vi "Drums with Guitar.vi"() -> ()   [LabVIEW 2009]
uses:
  <vilib>/vision/Image Controls.llb/IMAQ Image.ctl
  <vilib>/Instr/_visa.llb/VISA Configure Serial Port (Instr).vi
  <vilib>/Analysis/3filter.llb/Filter Passband Type.ctl
  <vilib>/Analysis/3filter.llb/Butterworth Filter (DBL).vi
  <vilib>/vision/NI_Vision_Development_Module.lvlib
  <vilib>/Analysis/NI_AALBase.lvlib
panel:
  in  "Orange Guitar":T1={"Global Rectangle"=[220, 296, 225, 371], "Contours"=[{"ID"=enum."External", "Type"=2, "Coordinates"=[224, 370, 220, 296]}]} {"Contours"."Type" items=["No Selection", "Point", "Line", "Rectangle", "Oval", "Polygon", "Freehand Region", "Annulus", "Unused2", "Unused3", "Broken Line", "Freehand Line", "Rotated Rectangle"]}
  out "Orange Guitar":dbl[](graph)
  out "Orange Guitar LED":bool
  in  "sampling 8":dbl=1.0 format="%0.2f"
  in  "high 9":dbl=60.0 format="%0.2f"
  in  "low  8":dbl=0.12500000000000006 format="%0.4f"
  out "Orange Guitar":T1={"Global Rectangle"=[300, 297, 320, 380], "Contours"=[{"ID"=enum."External", "Type"=2, "Coordinates"=[300, 379, 319, 297]}]} {"Contours"."Type" items=["No Selection", "Point", "Line", "Rectangle", "Oval", "Polygon", "Freehand Region", "Annulus", "Unused2", "Unused3", "Broken Line", "Freehand Line", "Rotated Rectangle"]}
  in  "Green Guitar":T1={"Global Rectangle"=[100, 292, 131, 371], "Contours"=[{"ID"=enum."External", "Type"=2, "Coordinates"=[100, 370, 130, 292]}]} {"Contours"."Type" items=["No Selection", "Point", "Line", "Rectangle", "Oval", "Polygon", "Freehand Region", "Annulus", "Unused2", "Unused3", "Broken Line", "Freehand Line", "Rotated Rectangle"]}
  in  "Blue Guitar":T1={"Global Rectangle"=[193, 293, 199, 374], "Contours"=[{"ID"=enum."External", "Type"=2, "Coordinates"=[193, 373, 198, 293]}]} {"Contours"."Type" items=["No Selection", "Point", "Line", "Rectangle", "Oval", "Polygon", "Freehand Region", "Annulus", "Unused2", "Unused3", "Broken Line", "Freehand Line", "Rotated Rectangle"]}
  in  "Red Guitar":T1={"Global Rectangle"=[129, 294, 154, 376], "Contours"=[{"ID"=enum."External", "Type"=2, "Coordinates"=[129, 375, 153, 294]}]} {"Contours"."Type" items=["No Selection", "Point", "Line", "Rectangle", "Oval", "Polygon", "Freehand Region", "Annulus", "Unused2", "Unused3", "Broken Line", "Freehand Line", "Rotated Rectangle"]}
  in  "Yellow Guitar":T1={"Global Rectangle"=[160, 295, 175, 378], "Contours"=[{"ID"=enum."External", "Type"=2, "Coordinates"=[160, 377, 174, 295]}]} {"Contours"."Type" items=["No Selection", "Point", "Line", "Rectangle", "Oval", "Polygon", "Freehand Region", "Annulus", "Unused2", "Unused3", "Broken Line", "Freehand Line", "Rotated Rectangle"]}
  in  "sampling  8":dbl=1.0 format="%0.2f"
  in  "high 8":dbl=60.0 format="%0.2f"
  out "Blue Guitar":dbl[](graph)
  in  "low 2":dbl=0.12500000000000006 format="%0.4f"
  out "Yellow Guitar":dbl[](graph)
  out "Yellow Guitar LED":bool
  in  "sampling 7":dbl=1.0 format="%0.2f"
  in  "high 7":dbl=60.0 format="%0.2f"
  in  "low  7":dbl=0.12500000000000006 format="%0.4f"
  out "Yellow Guitar":T1={"Global Rectangle"=[243, 262, 261, 384], "Contours"=[{"ID"=enum."External", "Type"=2, "Coordinates"=[260, 383, 243, 262]}]} {"Contours"."Type" items=["No Selection", "Point", "Line", "Rectangle", "Oval", "Polygon", "Freehand Region", "Annulus", "Unused2", "Unused3", "Broken Line", "Freehand Line", "Rotated Rectangle"]}
  out "Blue Guitar":T1={"Global Rectangle"=[168, 264, 180, 378], "Contours"=[{"ID"=enum."External", "Type"=2, "Coordinates"=[168, 377, 179, 264]}]} {"Contours"."Type" items=["No Selection", "Point", "Line", "Rectangle", "Oval", "Polygon", "Freehand Region", "Annulus", "Unused2", "Unused3", "Broken Line", "Freehand Line", "Rotated Rectangle"]}
  out "Green Guitar":dbl[](graph)
  out "Green Guitar LED":bool
  in  "sampling 6":dbl=1.0 format="%0.2f"
  in  "high 6":dbl=60.0 format="%0.2f"
  in  "low  6":dbl=0.12500000000000006 format="%0.4f"
  out "Green Guitar":T1={"Global Rectangle"=[406, 309, 423, 383], "Contours"=[{"ID"=enum."External", "Type"=2, "Coordinates"=[422, 382, 406, 309]}]} {"Contours"."Type" items=["No Selection", "Point", "Line", "Rectangle", "Oval", "Polygon", "Freehand Region", "Annulus", "Unused2", "Unused3", "Broken Line", "Freehand Line", "Rotated Rectangle"]}
  out "Red Guitar":dbl[](graph)
  out "Red Guitar LED":bool
  in  "sampling 5":dbl=1.0 format="%0.2f"
  in  "high 5":dbl=60.0 format="%0.2f"
  in  "low  5":dbl=0.12500000000000006 format="%0.4f"
  out "Red Guitar":T1={"Global Rectangle"=[300, 297, 320, 380], "Contours"=[{"ID"=enum."External", "Type"=2, "Coordinates"=[300, 379, 319, 297]}]} {"Contours"."Type" items=["No Selection", "Point", "Line", "Rectangle", "Oval", "Polygon", "Freehand Region", "Annulus", "Unused2", "Unused3", "Broken Line", "Freehand Line", "Rotated Rectangle"]}
  out "Blue Guitar LED":bool
  in  "Mask":T1 {"Contours"."Type" items=["No Selection", "Point", "Line", "Rectangle", "Oval", "Polygon", "Freehand Region", "Annulus", "Unused2", "Unused3", "Broken Line", "Freehand Line", "Rotated Rectangle"]}
  out "Image 2":T2(plugin-control)
  out "Red Line":T1={"Global Rectangle"=[300, 297, 320, 380], "Contours"=[{"ID"=enum."External", "Type"=2, "Coordinates"=[300, 379, 319, 297]}]} {"Contours"."Type" items=["No Selection", "Point", "Line", "Rectangle", "Oval", "Polygon", "Freehand Region", "Annulus", "Unused2", "Unused3", "Broken Line", "Freehand Line", "Rotated Rectangle"]}
  in  "Red Line":T1={"Global Rectangle"=[300, 297, 320, 380], "Contours"=[{"ID"=enum."External", "Type"=2, "Coordinates"=[300, 379, 319, 297]}]} {"Contours"."Type" items=["No Selection", "Point", "Line", "Rectangle", "Oval", "Polygon", "Freehand Region", "Annulus", "Unused2", "Unused3", "Broken Line", "Freehand Line", "Rotated Rectangle"]}
  out "Waveform Red":dbl[](graph)
  out "LED Red":bool
  in  "sampling 4":dbl=1.0 format="%0.2f"
  in  "high 4":dbl=60.0 format="%0.2f"
  in  "low  4":dbl=0.12500000000000006 format="%0.4f"
  out "Green Line":T1={"Global Rectangle"=[406, 309, 423, 383], "Contours"=[{"ID"=enum."External", "Type"=2, "Coordinates"=[422, 382, 406, 309]}]} {"Contours"."Type" items=["No Selection", "Point", "Line", "Rectangle", "Oval", "Polygon", "Freehand Region", "Annulus", "Unused2", "Unused3", "Broken Line", "Freehand Line", "Rotated Rectangle"]}
  in  "Blue Line":T1={"Global Rectangle"=[374, 278, 383, 377], "Contours"=[{"ID"=enum."External", "Type"=2, "Coordinates"=[382, 376, 374, 278]}]} {"Contours"."Type" items=["No Selection", "Point", "Line", "Rectangle", "Oval", "Polygon", "Freehand Region", "Annulus", "Unused2", "Unused3", "Broken Line", "Freehand Line", "Rotated Rectangle"]}
  in  "Green Line":T1={"Global Rectangle"=[406, 309, 423, 383], "Contours"=[{"ID"=enum."External", "Type"=2, "Coordinates"=[422, 382, 406, 309]}]} {"Contours"."Type" items=["No Selection", "Point", "Line", "Rectangle", "Oval", "Polygon", "Freehand Region", "Annulus", "Unused2", "Unused3", "Broken Line", "Freehand Line", "Rotated Rectangle"]}
  in  "low  3":dbl=0.12500000000000006 format="%0.4f"
  out "Waveform Green":dbl[](graph)
  out "LED Green":bool
  in  "sampling 3":dbl=1.0 format="%0.2f"
  in  "high 3":dbl=60.0 format="%0.2f"
  in  "Yellow Line":T1={"Global Rectangle"=[342, 292, 349, 377], "Contours"=[{"ID"=enum."External", "Type"=2, "Coordinates"=[342, 376, 348, 292]}]} {"Contours"."Type" items=["No Selection", "Point", "Line", "Rectangle", "Oval", "Polygon", "Freehand Region", "Annulus", "Unused2", "Unused3", "Broken Line", "Freehand Line", "Rotated Rectangle"]}
  out "Blue Line":T1={"Global Rectangle"=[168, 264, 180, 378], "Contours"=[{"ID"=enum."External", "Type"=2, "Coordinates"=[168, 377, 179, 264]}]} {"Contours"."Type" items=["No Selection", "Point", "Line", "Rectangle", "Oval", "Polygon", "Freehand Region", "Annulus", "Unused2", "Unused3", "Broken Line", "Freehand Line", "Rotated Rectangle"]}
  out "cluster":T3
  in  "baud rate (9600)":u32=9600
  in  "VISA resource name":refnum<visa-resource-name>
  out "number":u32
  out "decimal integer string":string
  out "Image Dst Out":T2
  out "Yellow Line":T1={"Global Rectangle"=[243, 262, 261, 384], "Contours"=[{"ID"=enum."External", "Type"=2, "Coordinates"=[260, 383, 243, 262]}]} {"Contours"."Type" items=["No Selection", "Point", "Line", "Rectangle", "Oval", "Polygon", "Freehand Region", "Annulus", "Unused2", "Unused3", "Broken Line", "Freehand Line", "Rotated Rectangle"]}
  in  "low  2":dbl=0.12500000000000006 format="%0.4f"
  in  "high 2":dbl=60.0 format="%0.2f"
  in  "sampling 2":dbl=1.0 format="%0.2f"
  out "LED Yellow":bool
  out "Waveform Yellow":dbl[](graph)
  in  "playtime":dbl=30.0
  out "Frame Number":i32
  in  "Frame Start":i32=2400
  out "Blue Drum":bool
  in  "low":dbl=0.12500000000000006 format="%0.4f"
  out "Blue Drum":dbl[](graph)
  in  "high":dbl=60.0 format="%0.2f"
  in  "sampling":dbl=1.0 format="%0.2f"
  in  "stop":bool
  in  "AVI Path":path
  # "BLUE"
  # "YELLOW"
  # "GREEN"
  # "RED"
  # "Drums"
  # "Guitar"
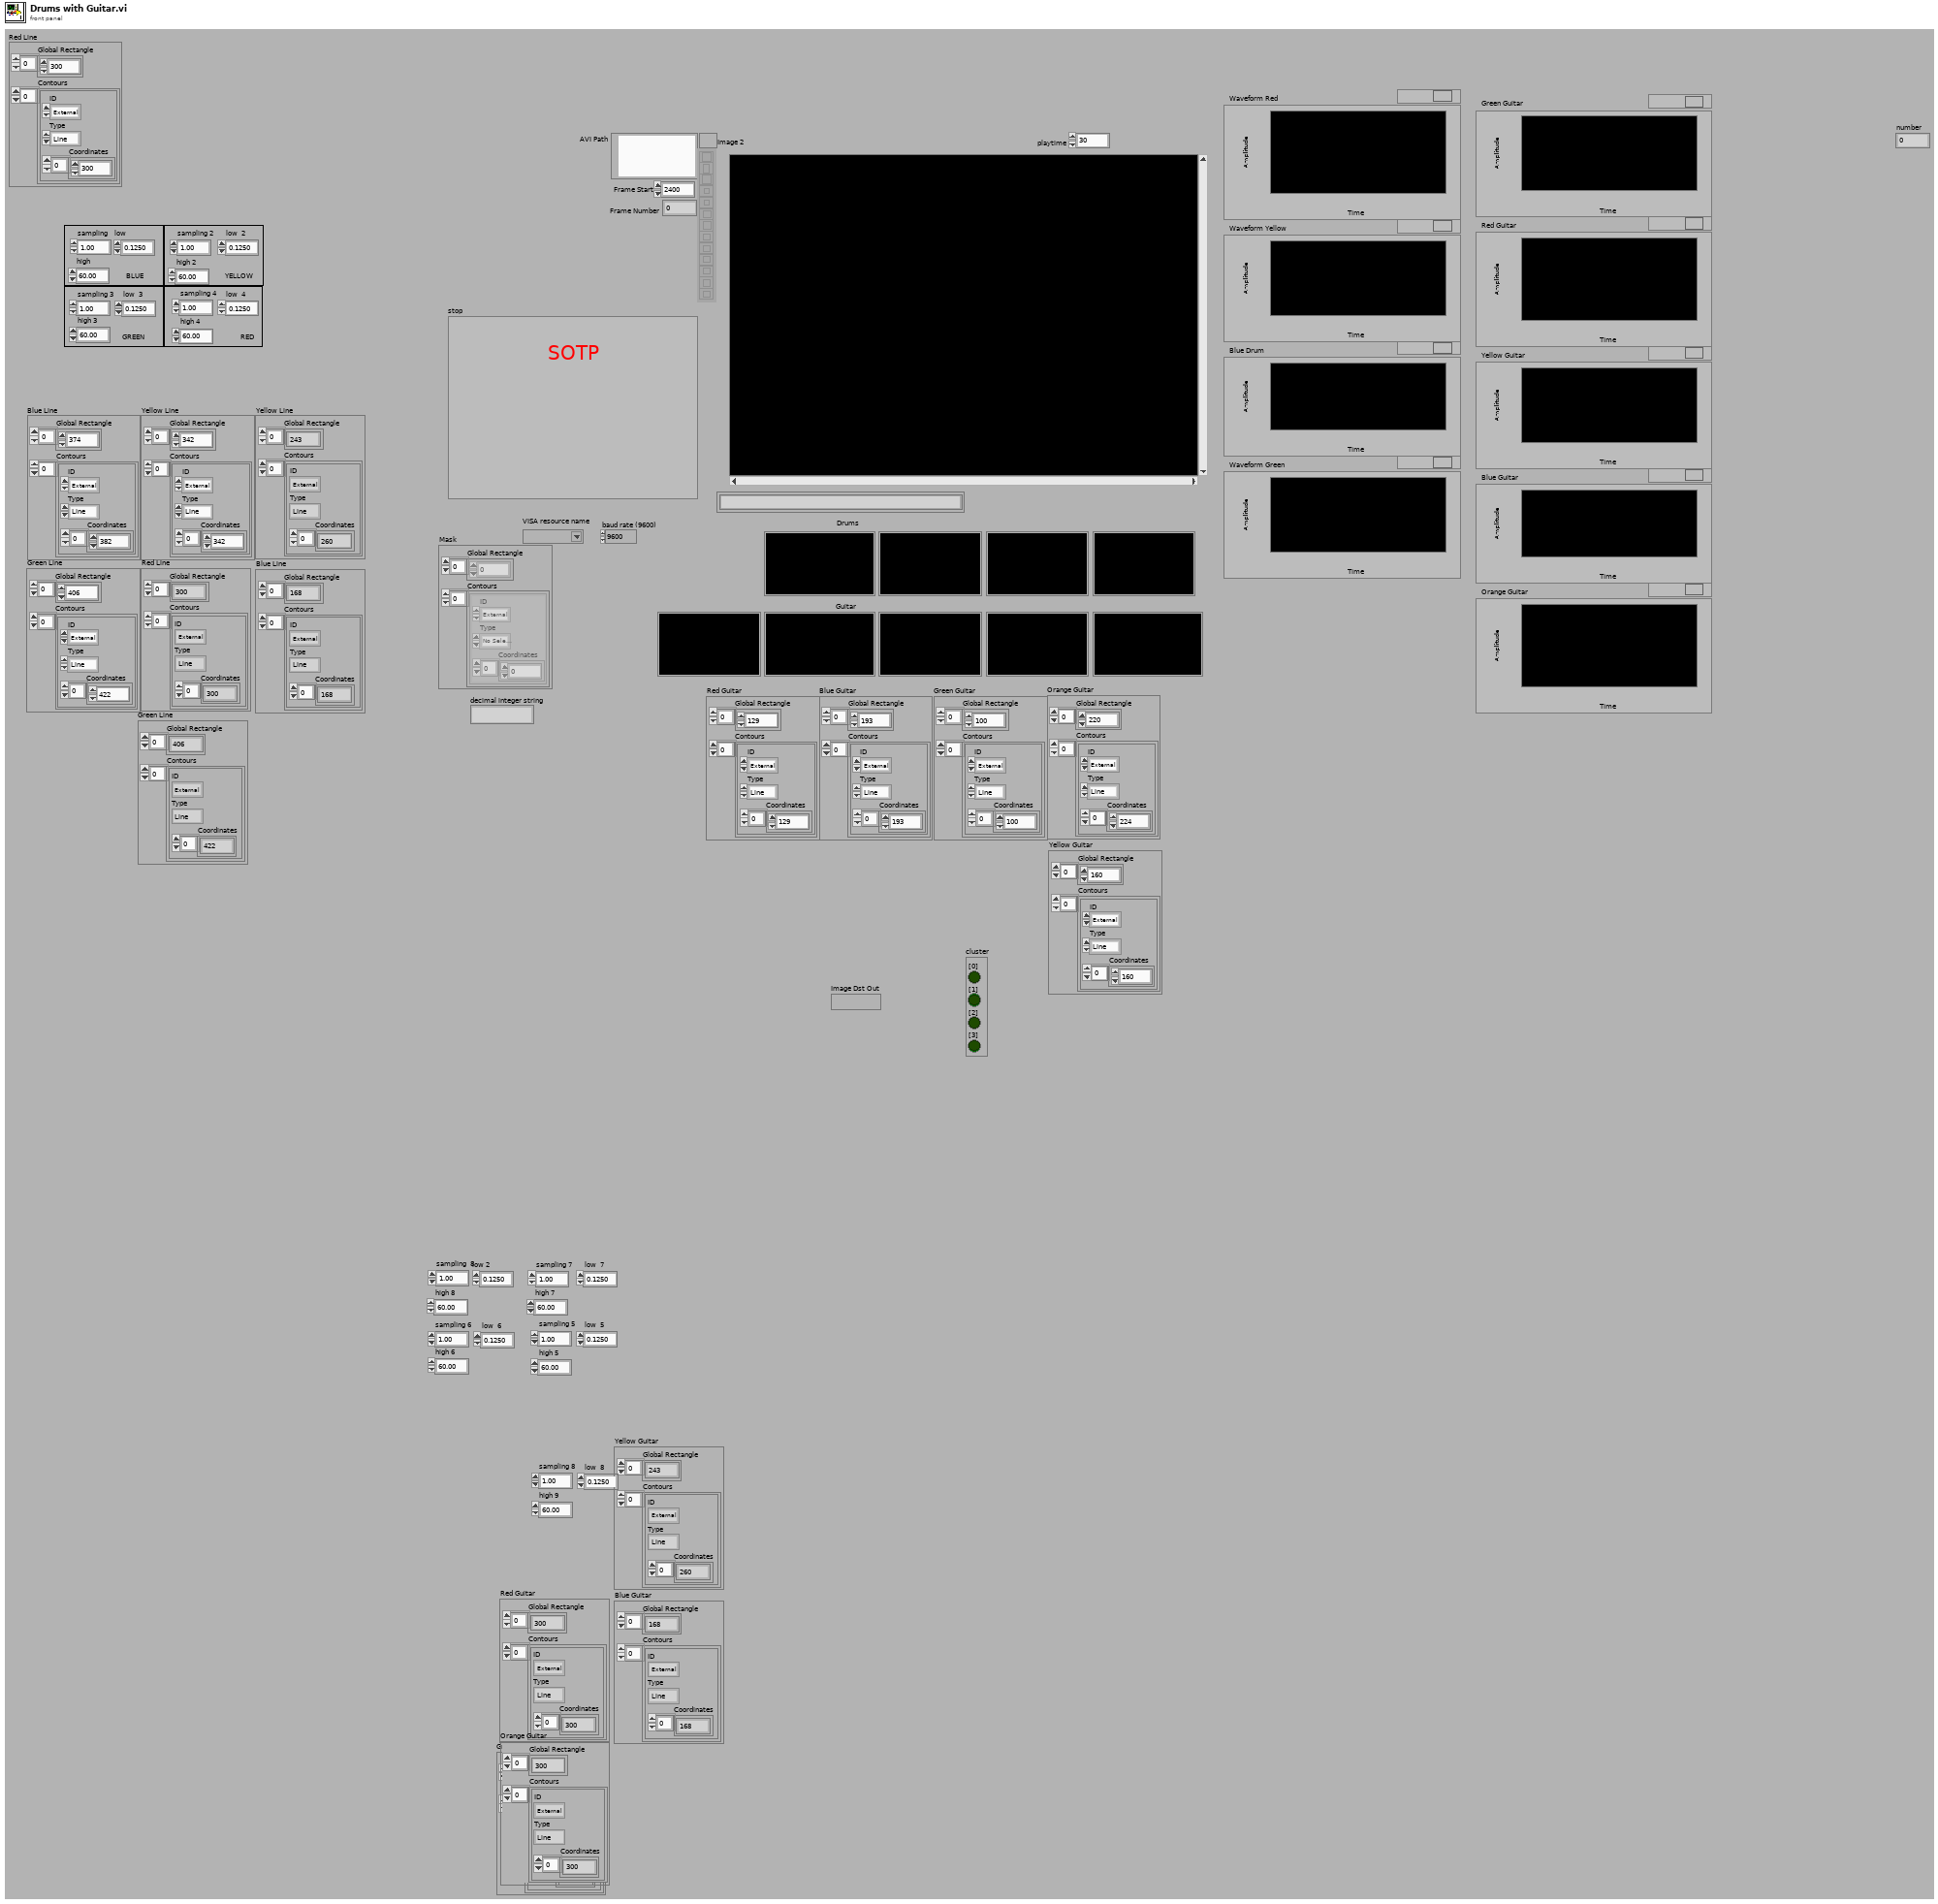
[diagram p1: front panel]
types:
  T1 = cluster{"Global Rectangle":i32[], "Contours":cluster{"ID":enum32{"External", "Internal"}, "Type":u32, "Coordinates":i32[]}[]}
  T2 = typedef "IMAQ Image.ctl" = refnum<image>
  T3 = cluster{"[0]":bool, "[1]":bool, "[2]":bool, "[3]":bool, "[4]":bool, "[5]":bool, "[6]":bool, "[7]":bool, "[8]":bool}
  T4 = typedef "NI_AALBase.lvlib/Filter Passband Type.ctl" = enum32{"Lowpass", "Highpass", "Bandpass", "Bandstop"}
  T5 = cluster{"Left":i32, "Top":i32, "Right":i32, "Bottom":i32}
  T6 = typedef "Image Type" = u32
  T7 = typedef "AviRefnum.ctl" = refnum<k1>
  T8 = cluster{"ID":enum32{"External", "Internal"}, "Type":u32, "Coordinates":i32[]}[]
  T9 = cluster{"ID":enum32{"External", "Internal"}, "Type":u32, "Coordinates":i32[]}
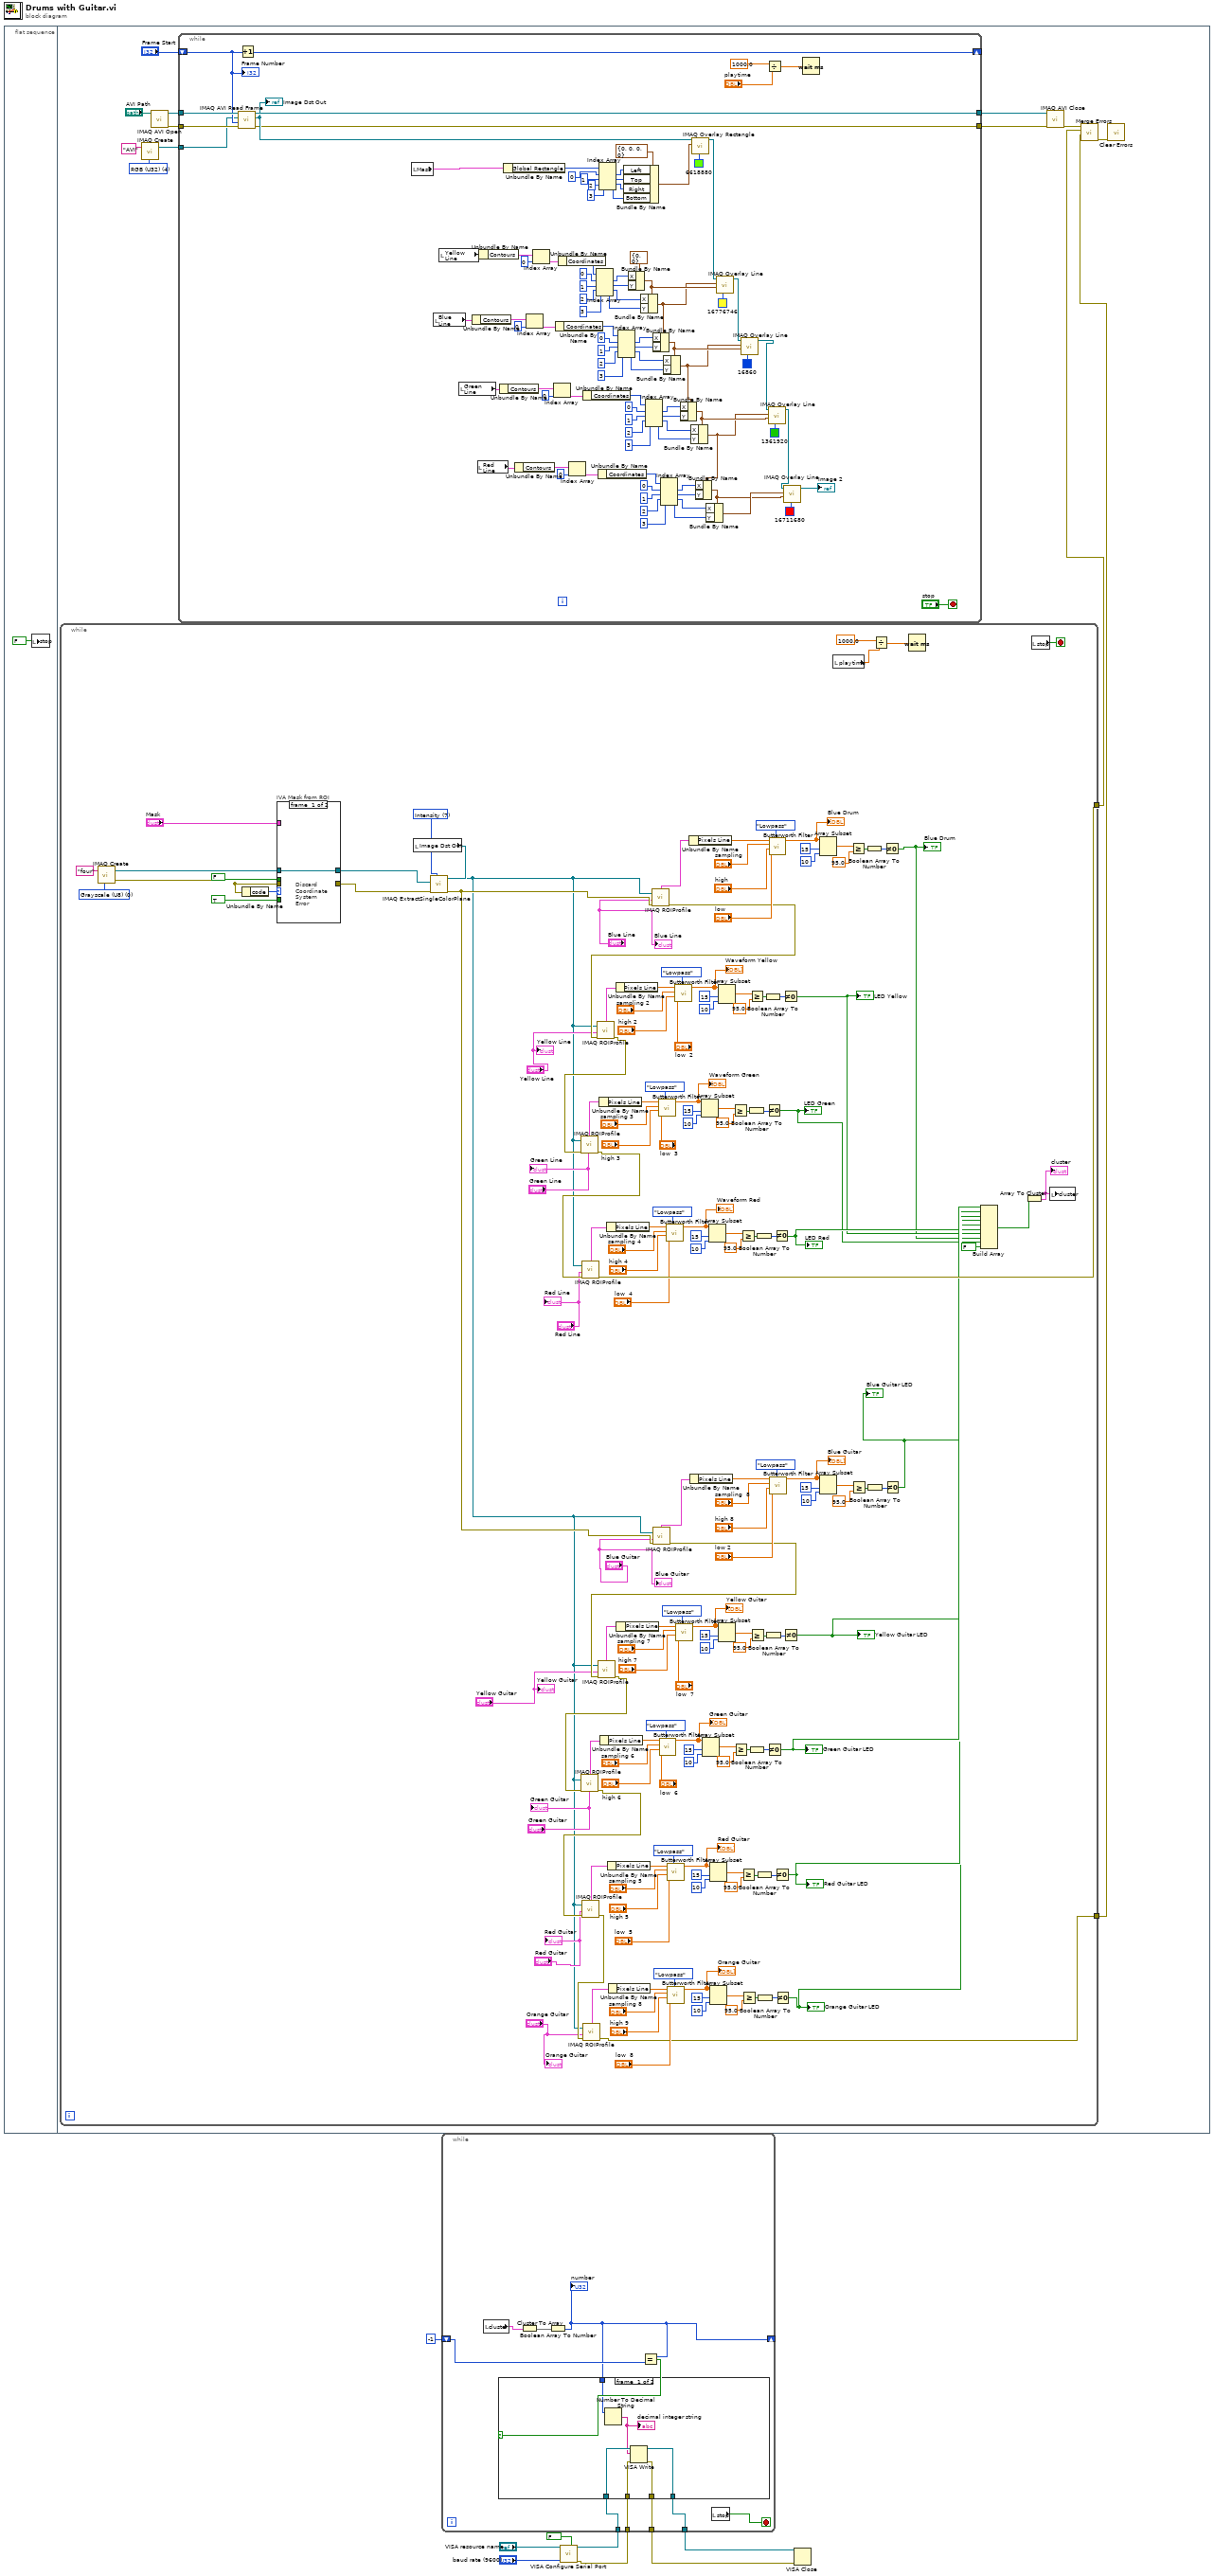
[diagram p0: block diagram]
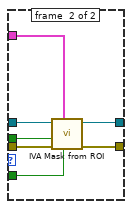
[diagram p3: hidden frame]
diagram:
  n1 = flat-sequence {
    frame #0 {
      n2 = local write "stop"(FALSE ("stop")) -> ()
    }
    frame #1 {
      w14 = T6 4 items=["Grayscale (U8)", "Grayscale (I16)", "Grayscale (SGL)", "Complex (CSG)", "RGB (U32)", "HSL (U32)", "RGB (U64)", "Grayscale (U16)"] ("Image Type")
      n3 = while {
        tunnel: [w171] -> w11
        tunnel: [w35] -> w10
        stop <- w186 stop-if-true
        w181 = T6 0 items=["Grayscale (U8)", "Grayscale (I16)", "Grayscale (SGL)", "Complex (CSG)", "RGB (U32)", "HSL (U32)", "RGB (U64)", "Grayscale (U16)"] ("Image Type")
        w187 = 7 items=["Red", "Green", "Blue", "Hue", "Saturation", "Luminance", "Value", "Intensity"] ("Color Plane")
        n4 = call "IMAQ Create"("Image Name"="four", "Image Type"=w181) -> ("New Image"=w174:T2, "error out"=w175:errorcluster)  [unwired: 3 in]
        n5 = Unbundle By Name(w175) -> ("code"=w179:i32)
        n6 = case "IVA Mask from ROI" shown="Default" w179 {
          tunnel: "Mask" -> [_ w195]
          tunnel: TRUE ("Shrink") -> [_ w194]
          tunnel: w174 -> [w188 w193]
          tunnel: w175 -> [_ w192]
          tunnel: [_ w191] -> w176
          tunnel: [w188 w190] -> w172
          tunnel: FALSE ("Out / In") -> [_ w189]
          frame #0 {
            # "Discard\nCoordinate\nSystem\nError"
          }
          frame #1 {
            n7 = call <vilib>:"IVA Mask from ROI.vi"("Shrink"=w194, "ROI Descriptor"=w195, "error in (no error)"=w192, "Out / In"=w189, "Image Src"=w193) -> ("error out"=w191:errorcluster, "Image Out"=w190:T2)  [unwired: 5 out]
          }
        }
        n8 = local read "Image Dst Out"() -> (w182:T2)
        n9 = call "IMAQ ExtractSingleColorPlane"("Color Plane"=w187, "error in (no error)"=w176, "Image Dst"=w172, "Image Src"=w182) -> ("error out"=w170:errorcluster, "Image Dst Out"=w34:T2)  [unwired: 6 out]
        n10 = call "IMAQ ROIProfile"("error in (no error)"=w170, "ROI Descriptor"="Blue Line", "Image"=w34) -> ("error out"=w145:errorcluster, "ROI Graph"=w144:cluster{"x0":sgl, "dx":sgl, "Pixels Line":sgl[]})  [unwired: 4 out]
        n11 = call "IMAQ ROIProfile"("error in (no error)"=w145, "ROI Descriptor"="Yellow Line", "Image"=w34) -> ("error out"=w112:errorcluster, "ROI Graph"=w148:cluster{"x0":sgl, "dx":sgl, "Pixels Line":sgl[]})  [unwired: 4 out]
        n12 = call "IMAQ ROIProfile"("error in (no error)"=w112, "ROI Descriptor"="Green Line", "Image"=w34) -> ("error out"=w115:errorcluster, "ROI Graph"=w142:cluster{"x0":sgl, "dx":sgl, "Pixels Line":sgl[]})  [unwired: 4 out]
        n13 = call "IMAQ ROIProfile"("error in (no error)"=w115, "ROI Descriptor"="Red Line", "Image"=w34) -> ("error out"=w171:errorcluster, "ROI Graph"=w117:cluster{"x0":sgl, "dx":sgl, "Pixels Line":sgl[]})  [unwired: 4 out]
        n14 = Unbundle By Name(w142) -> ("Pixels Line"=w139:sgl[])
        n15 = Unbundle By Name(w117) -> ("Pixels Line"=w120:sgl[])
        n16 = Unbundle By Name(w148) -> ("Pixels Line"=w151:sgl[])
        n17 = call "IMAQ ROIProfile"("error in (no error)"=w170, "ROI Descriptor"="Blue Guitar", "Image"=w34) -> ("error out"=w84:errorcluster, "ROI Graph"=w83:cluster{"x0":sgl, "dx":sgl, "Pixels Line":sgl[]})  [unwired: 4 out]
        n18 = call "IMAQ ROIProfile"("error in (no error)"=w84, "ROI Descriptor"="Yellow Guitar", "Image"=w34) -> ("error out"=w54:errorcluster, "ROI Graph"=w87:cluster{"x0":sgl, "dx":sgl, "Pixels Line":sgl[]})  [unwired: 4 out]
        n19 = call "IMAQ ROIProfile"("error in (no error)"=w54, "ROI Descriptor"="Green Guitar", "Image"=w34) -> ("error out"=w55:errorcluster, "ROI Graph"=w81:cluster{"x0":sgl, "dx":sgl, "Pixels Line":sgl[]})  [unwired: 4 out]
        n20 = call "IMAQ ROIProfile"("error in (no error)"=w55, "ROI Descriptor"="Red Guitar", "Image"=w34) -> ("error out"=w36:errorcluster, "ROI Graph"=w57:cluster{"x0":sgl, "dx":sgl, "Pixels Line":sgl[]})  [unwired: 4 out]
        n21 = call "IMAQ ROIProfile"("error in (no error)"=w36, "ROI Descriptor"="Orange Guitar", "Image"=w34) -> ("error out"=w35:errorcluster, "ROI Graph"=w48:cluster{"x0":sgl, "dx":sgl, "Pixels Line":sgl[]})  [unwired: 4 out]
        n22 = Unbundle By Name(w81) -> ("Pixels Line"=w78:sgl[])
        n23 = Unbundle By Name(w57) -> ("Pixels Line"=w60:sgl[])
        n24 = Unbundle By Name(w48) -> ("Pixels Line"=w45:sgl[])
        n25 = Unbundle By Name(w87) -> ("Pixels Line"=w90:sgl[])
        n26 = call-poly <vilib>:"Butterworth Filter.vi"("filter type"=Filter_Passband_Type."Lowpass", "low cutoff freq: fl"="low  3", "high cutoff freq: fh"="high 3", "sampling freq: fs"="sampling 3", "X"=w139) -> ("Filtered X"=w143:dbl[])  [unwired: 3 in, 1 out]
        "Waveform Green" <- w143
        n27 = call-poly <vilib>:"Butterworth Filter.vi"("filter type"=Filter_Passband_Type."Lowpass", "low cutoff freq: fl"="low  6", "high cutoff freq: fh"="high 6", "sampling freq: fs"="sampling 6", "X"=w78) -> ("Filtered X"=w82:dbl[])  [unwired: 3 in, 1 out]
        "Green Guitar" <- w82
        n28 = call-poly <vilib>:"Butterworth Filter.vi"("filter type"=Filter_Passband_Type."Lowpass", "low cutoff freq: fl"="low  4", "high cutoff freq: fh"="high 4", "sampling freq: fs"="sampling 4", "X"=w120) -> ("Filtered X"=w116:dbl[])  [unwired: 3 in, 1 out]
        "Waveform Red" <- w116
        n29 = call-poly <vilib>:"Butterworth Filter.vi"("filter type"=Filter_Passband_Type."Lowpass", "low cutoff freq: fl"="low  5", "high cutoff freq: fh"="high 5", "sampling freq: fs"="sampling 5", "X"=w60) -> ("Filtered X"=w56:dbl[])  [unwired: 3 in, 1 out]
        "Red Guitar" <- w56
        n30 = call-poly <vilib>:"Butterworth Filter.vi"("filter type"=Filter_Passband_Type."Lowpass", "low cutoff freq: fl"="low  8", "high cutoff freq: fh"="high 9", "sampling freq: fs"="sampling 8", "X"=w45) -> ("Filtered X"=w49:dbl[])  [unwired: 3 in, 1 out]
        "Orange Guitar" <- w49
        n31 = call-poly <vilib>:"Butterworth Filter.vi"("filter type"=Filter_Passband_Type."Lowpass", "low cutoff freq: fl"="low  2", "high cutoff freq: fh"="high 2", "sampling freq: fs"="sampling 2", "X"=w151) -> ("Filtered X"=w147:dbl[])  [unwired: 3 in, 1 out]
        "Waveform Yellow" <- w147
        n32 = call-poly <vilib>:"Butterworth Filter.vi"("filter type"=Filter_Passband_Type."Lowpass", "low cutoff freq: fl"="low  7", "high cutoff freq: fh"="high 7", "sampling freq: fs"="sampling 7", "X"=w90) -> ("Filtered X"=w86:dbl[])  [unwired: 3 in, 1 out]
        "Yellow Guitar" <- w86
        n33 = Unbundle By Name(w144) -> ("Pixels Line"=w168:sgl[])
        n34 = Unbundle By Name(w83) -> ("Pixels Line"=w107:sgl[])
        n35 = Array Subset(array=w143, index=15, length=10) -> (w134:dbl[])
        n36 = Array Subset(array=w82, index=15, length=10) -> (w73:dbl[])
        n37 = Array Subset(array=w116, index=15, length=10) -> (w125:dbl[])
        n38 = Array Subset(array=w56, index=15, length=10) -> (w65:dbl[])
        n39 = Array Subset(array=w49, index=15, length=10) -> (w40:dbl[])
        n40 = Array Subset(array=w147, index=15, length=10) -> (w156:dbl[])
        n41 = Array Subset(array=w86, index=15, length=10) -> (w95:dbl[])
        n42 = Greater Or Equal?(x=w134, y=95.0) -> (x >= y?=w136:bool[])
        n43 = Greater Or Equal?(x=w73, y=95.0) -> (x >= y?=w75:bool[])
        n44 = Greater Or Equal?(x=w125, y=95.0) -> (x >= y?=w123:bool[])
        n45 = Greater Or Equal?(x=w65, y=95.0) -> (x >= y?=w63:bool[])
        n46 = Greater Or Equal?(x=w40, y=95.0) -> (x >= y?=w42:bool[])
        n47 = Boolean Array To Number(Boolean array=w136) -> (number=w137:u32)
        n48 = Greater Or Equal?(x=w156, y=95.0) -> (x >= y?=w154:bool[])
        n49 = Boolean Array To Number(Boolean array=w75) -> (number=w76:u32)
        n50 = Greater Or Equal?(x=w95, y=95.0) -> (x >= y?=w93:bool[])
        n51 = Boolean Array To Number(Boolean array=w123) -> (number=w122:u32)
        n52 = Boolean Array To Number(Boolean array=w63) -> (number=w62:u32)
        n53 = Boolean Array To Number(Boolean array=w42) -> (number=w43:u32)
        n54 = Boolean Array To Number(Boolean array=w154) -> (number=w153:u32)
        n55 = Boolean Array To Number(Boolean array=w93) -> (number=w92:u32)
        n56 = Not Equal To 0?(x=w137) -> (x != 0?=w24:bool)
        "LED Green" <- w24
        n57 = Not Equal To 0?(x=w76) -> (x != 0?=w32:bool)
        "Green Guitar LED" <- w32
        n58 = call-poly <vilib>:"Butterworth Filter.vi"("filter type"=Filter_Passband_Type."Lowpass", "low cutoff freq: fl"="low", "high cutoff freq: fh"="high", "sampling freq: fs"="sampling", "X"=w168) -> ("Filtered X"=w130:dbl[])  [unwired: 3 in, 1 out]
        "Blue Drum" <- w130
        n59 = call-poly <vilib>:"Butterworth Filter.vi"("filter type"=Filter_Passband_Type."Lowpass", "low cutoff freq: fl"="low 2", "high cutoff freq: fh"="high 8", "sampling freq: fs"="sampling  8", "X"=w107) -> ("Filtered X"=w69:dbl[])  [unwired: 3 in, 1 out]
        "Blue Guitar" <- w69
        n60 = Not Equal To 0?(x=w122) -> (x != 0?=w27:bool)
        "LED Red" <- w27
        n61 = Not Equal To 0?(x=w62) -> (x != 0?=w31:bool)
        "Red Guitar LED" <- w31
        n62 = Not Equal To 0?(x=w43) -> (x != 0?=w28:bool)
        "Orange Guitar LED" <- w28
        n63 = Not Equal To 0?(x=w153) -> (x != 0?=w26:bool)
        "LED Yellow" <- w26
        n64 = Not Equal To 0?(x=w92) -> (x != 0?=w30:bool)
        "Yellow Guitar LED" <- w30
        n65 = Array Subset(array=w130, index=15, length=10) -> (w162:dbl[])
        n66 = Array Subset(array=w69, index=15, length=10) -> (w101:dbl[])
        n67 = local read "playtime"() -> (w183:dbl)
        n68 = Greater Or Equal?(x=w162, y=95.0) -> (x >= y?=w160:bool[])
        n69 = Greater Or Equal?(x=w101, y=95.0) -> (x >= y?=w99:bool[])
        n70 = Boolean Array To Number(Boolean array=w160) -> (number=w159:u32)
        n71 = Boolean Array To Number(Boolean array=w99) -> (number=w98:u32)
        n72 = Divide(x=1000.0, y=w183) -> (x/y=w185:dbl)
        n73 = Not Equal To 0?(x=w159) -> (x != 0?=w25:bool)
        "Blue Drum" <- w25
        n74 = Not Equal To 0?(x=w98) -> (x != 0?=w29:bool)
        "Blue Guitar LED" <- w29
        n75 = Wait (ms)(milliseconds to wait=w185) -> ()  [unwired: 1 out]
        n76 = Build Array(w32, w31, w30, w29, w28, w27, w26, w25, w24, FALSE ("element")) -> (w110:bool[])
        n77 = Array To Cluster(array=w110) -> (cluster=w111:T3)
        "cluster" <- w111
        n78 = local read "stop"() -> (w186:bool)
        n79 = local write "cluster"(w111) -> ()
        "Yellow Line" <- "Yellow Line"
        "Blue Line" <- "Blue Line"
        "Green Line" <- "Green Line"
        "Red Line" <- "Red Line"
        "Yellow Guitar" <- "Yellow Guitar"
        "Blue Guitar" <- "Blue Guitar"
        "Green Guitar" <- "Green Guitar"
        "Red Guitar" <- "Red Guitar"
        "Orange Guitar" <- "Orange Guitar"
      }
      n80 = call "IMAQ Create"("Image Name"="AVI", "Image Type"=w14) -> ("New Image"=w12:T2)  [unwired: 3 in, 1 out]
      n81 = call "IMAQ AVI Open"("AVI Path"="AVI Path") -> ("error out"=w19:errorcluster, "Avi Refnum"=w20:T7)  [unwired: 9 in]
      n82 = while {
        tunnel: w20 -> [w290]
        tunnel: w19 -> [w238]
        tunnel: [w289] -> w21
        shift-right: [w284] -> _
        shift-left: "Frame Start" -> [w283]
        tunnel: [w234] -> w15
        tunnel: w12 -> [w233]
        stop <- "stop" stop-if-true
        n83 = call "IMAQ AVI Read Frame"("error in (no error)"=w238, "Frame Number"=w283, "Image"=w233, "Avi Refnum"=w290) -> ("error out"=w234:errorcluster, "Image Out"=w235:T2, "Avi Refnum (duplicate)"=w289:T7)  [unwired: 4 in, 1 out]
        "Image Dst Out" <- w235
        n84 = Increment(x=w283) -> (x+1=w284:i32)
        n85 = local read "Mask"() -> (w196:T1)
        n86 = local read "Blue Line"() -> (w237:T1)
        n87 = local read "Yellow Line"() -> (w236:T1)
        n88 = local read "Green Line"() -> (w232:T1)
        n89 = Unbundle By Name(w237) -> ("Contours"=w250:T8)
        n90 = local read "Red Line"() -> (w199:T1)
        n91 = Unbundle By Name(w236) -> ("Contours"=w265:T8)
        n92 = Unbundle By Name(w232) -> ("Contours"=w222:T8)
        n93 = Unbundle By Name(w196) -> ("Global Rectangle"=w279:i32[])
        n94 = Unbundle By Name(w199) -> ("Contours"=w209:T8)
        n95 = Index Array(array=w250, index=0) -> (element=w249:T9)
        n96 = Index Array(array=w265, index=0) -> (element=w267:T9)
        n97 = Index Array(array=w222, index=0) -> (element=w223:T9)
        n98 = Unbundle By Name(w249) -> ("Coordinates"=w248:i32[])
        n99 = Unbundle By Name(w267) -> ("Coordinates"=w268:i32[])
        n100 = Index Array(array=w209, index=0) -> (element=w208:T9)
        n101 = Unbundle By Name(w223) -> ("Coordinates"=w224:i32[])
        n102 = Index Array(array=w268, index #1=0 ("index"), index #2=1 ("index"), index #3=2 ("index"), index #4=3 ("index")) -> (element #1=w260:i32, element #2=w261:i32, element #3=w262:i32, element #4=w263:i32)
        n103 = Unbundle By Name(w208) -> ("Coordinates"=w207:i32[])
        n104 = Index Array(array=w279, index #1=0 ("index"), index #2=1 ("index"), index #3=2 ("index"), index #4=3 ("index")) -> (element #1=w278:i32, element #2=w277:i32, element #3=w276:i32, element #4=w275:i32)
        n105 = Index Array(array=w248, index #1=0 ("index"), index #2=1 ("index"), index #3=2 ("index"), index #4=3 ("index")) -> (element #1=w247:i32, element #2=w253:i32, element #3=w252:i32, element #4=w251:i32)
        n106 = Bundle By Name(cluster=T5 {"Left"=0, "Top"=0, "Right"=0, "Bottom"=0} ("Rectangle"), "Left"=w278, "Top"=w277, "Right"=w276, "Bottom"=w275) -> (w281:T5)
        n107 = Bundle By Name(cluster=cluster{"X":i32, "Y":i32} {"X"=0, "Y"=0} ("End Point"), "X"=w260, "Y"=w261) -> (w269:cluster{"X":i32, "Y":i32})
        n108 = Bundle By Name(cluster=w269, "X"=w262, "Y"=w263) -> (w240:cluster{"X":i32, "Y":i32})
        n109 = Index Array(array=w224, index #1=0 ("index"), index #2=1 ("index"), index #3=2 ("index"), index #4=3 ("index")) -> (element #1=w225:i32, element #2=w219:i32, element #3=w220:i32, element #4=w221:i32)
        n110 = Bundle By Name(cluster=w240, "X"=w247, "Y"=w253) -> (w254:cluster{"X":i32, "Y":i32})
        n111 = Index Array(array=w207, index #1=0 ("index"), index #2=1 ("index"), index #3=2 ("index"), index #4=3 ("index")) -> (element #1=w206:i32, element #2=w212:i32, element #3=w211:i32, element #4=w210:i32)
        n112 = Bundle By Name(cluster=w254, "X"=w252, "Y"=w251) -> (w217:cluster{"X":i32, "Y":i32})
        n113 = Bundle By Name(cluster=w217, "X"=w225, "Y"=w219) -> (w216:cluster{"X":i32, "Y":i32})
        n114 = Bundle By Name(cluster=w216, "X"=w220, "Y"=w221) -> (w198:cluster{"X":i32, "Y":i32})
        n115 = call "IMAQ Overlay Rectangle"("Color"=u32 6618880, "Rectangle"=w281, "Image"=w235) -> ("Image Out"=w255:T2)  [unwired: 7 in, 1 out]
        n116 = Bundle By Name(cluster=w198, "X"=w206, "Y"=w212) -> (w214:cluster{"X":i32, "Y":i32})
        n117 = Bundle By Name(cluster=w214, "X"=w211, "Y"=w210) -> (w215:cluster{"X":i32, "Y":i32})
        n118 = call "IMAQ Overlay Line"("Color"=u32 16776746, "End Point"=w269, "Start Point"=w240, "Image"=w255) -> ("Image Out"=w245:T2)  [unwired: 6 in, 1 out]
        n119 = call "IMAQ Overlay Line"("Color"=u32 16860, "End Point"=w254, "Start Point"=w217, "Image"=w245) -> ("Image Out"=w218:T2)  [unwired: 6 in, 1 out]
        n120 = Divide(x=1000.0, y="playtime") -> (x/y=w287:dbl)
        n121 = call "IMAQ Overlay Line"("Color"=u32 1361920, "End Point"=w216, "Start Point"=w198, "Image"=w218) -> ("Image Out"=w197:T2)  [unwired: 6 in, 1 out]
        n122 = call "IMAQ Overlay Line"("Color"=u32 16711680, "End Point"=w214, "Start Point"=w215, "Image"=w197) -> ("Image Out"=→"Image 2":T2)  [unwired: 6 in, 1 out]
        n123 = Wait (ms)(milliseconds to wait=w287) -> ()  [unwired: 1 out]
        "Frame Number" <- w283
      }
      n124 = call "IMAQ AVI Close"("error in (no error)"=w15, "Avi Refnum"=w21) -> ("error out"=w17:errorcluster)  [unwired: 9 in]
      n125 = call <vilib>:"Merge Errors.vi"("error in 3 (no error)"=w10, "error in 2 (no error)"=w11, "error in 1 (no error)"=w17) -> ("error out"=w16:errorcluster)  [unwired: 4 in]
      n126 = call <vilib>:"Clear Errors.vi"("error in (no error)"=w16) -> ()  [unwired: 6 in, 1 out]
    }
  }
  n127 = call-poly "VISA Configure Serial Port"("VISA resource name"="VISA resource name", "Enable Termination\nChar (T)"=FALSE ("Enable Termination\nChar (T)"), "baud rate (9600)"="baud rate (9600)") -> ("VISA resource name out"=w7:refnum<visa-resource-name>, "error out"=w2:errorcluster)  [unwired: 11 in]
  n128 = while {
    shift-right: [w294] -> _
    shift-left: -1 -> [w300]
    tunnel: w7 -> [w298]
    tunnel: [w297] -> w6
    tunnel: w2 -> [w296]
    tunnel: [w295] -> w1
    stop <- w291 stop-if-true
    n129 = local read "cluster"() -> (w292:T3)
    n130 = Cluster To Array(cluster=w292) -> (array=w293:bool[])
    n131 = Boolean Array To Number(Boolean array=w293) -> (number=w294:u32)
    "number" <- w294
    n132 = Equal?(x=w294, y=w300) -> (x = y?=w299:bool)
    n133 = case shown="False" w299 {
      tunnel: w298 -> [w306 w308]
      tunnel: [w305 w308] -> w297
      tunnel: w294 -> [w303 _]
      tunnel: w296 -> [w302 w307]
      tunnel: [w301 w307] -> w295
      frame #0 {
        n134 = Number To Decimal String(number=w303) -> (decimal integer string=w304:string)  [unwired: 1 in]
        "decimal integer string" <- w304
        n135 = VISA Write(VISA resource name=w306, write buffer=w304, error in (no error)=w302) -> (VISA resource name out=w305:refnum<visa-resource-name>, error out=w301:errorcluster)  [unwired: 1 out]
      }
      frame #1 {
      }
    }
    n136 = local read "stop"() -> (w291:bool)
  }
  n137 = VISA Close(VISA resource name=w6, error in (no error)=w1) -> ()  [unwired: 1 out]
